vi "Initialize FPGA.vi"() -> (3 "IO Cluster Out":T1={"Error"={"status"=FALSE, "code"=0, "source"=""}, "Encoder Calibration Values"=[22, 216], "Update Calibration"=FALSE, "JPEG Resolutions"=3, "Raw Resolutions"=1, "Image Mode"=enum."RAW Gray Scale", "FPGA Ref"=refnum} {"JPEG Resolutions" items=["160x128"=3, "320x240"=5, "640x480"=7]; "Raw Resolutions" items=["80x60"=1, "160x120"=3, "128x128"=9, "128x96"=11]})   [LabVIEW 2019]
uses:
  QNET MS IO Cluster.ctl
  <vilib>/FPGAPlugInAG/myRIO-1900/niLvFpga_Open_myRIO-1900.vi
  <vilib>/rvi/interface/common/dynamic/niFpgaDynamicAddResources.vi
  <vilib>/rvi/interface/common/niFpgaWaitOnOcc.vi
  <vilib>/Utility/error.llb/Error Cluster From Error Code.vi
  <vilib>/rvi/errors/niLvFpgaAdjustHostInterfaceError.vi
  <vilib>/rvi/interface/nirviOpenFPGA/nirviOpenFPGA.xnode
  <vilib>/rvi/interface/nirviMethod/nirviMethod.xnode
  <vilib>/rvi/interface/nirviReadWriteControl/nirviReadWriteControl.xnode
  <vilib>/ErrorRing/Error Ring.xnode
  <vilib>/FPGAPlugInAG/Dynamic/niLvFpga_ConfigureFifo_Dynamic.vi
  <vilib>/rvi/errors/niLvFpgaMergeErrorWithErrorCode.vi
  <vilib>/FPGAPlugInAG/Dynamic/niLvFpga_StartFifo_Dynamic.vi
  NiFpgaLv.dll
  <vilib>/rvi/interface/Simulation/niFpgaSimulationCallBeginRW.vi
panel:
  out "Actual Depth":u32
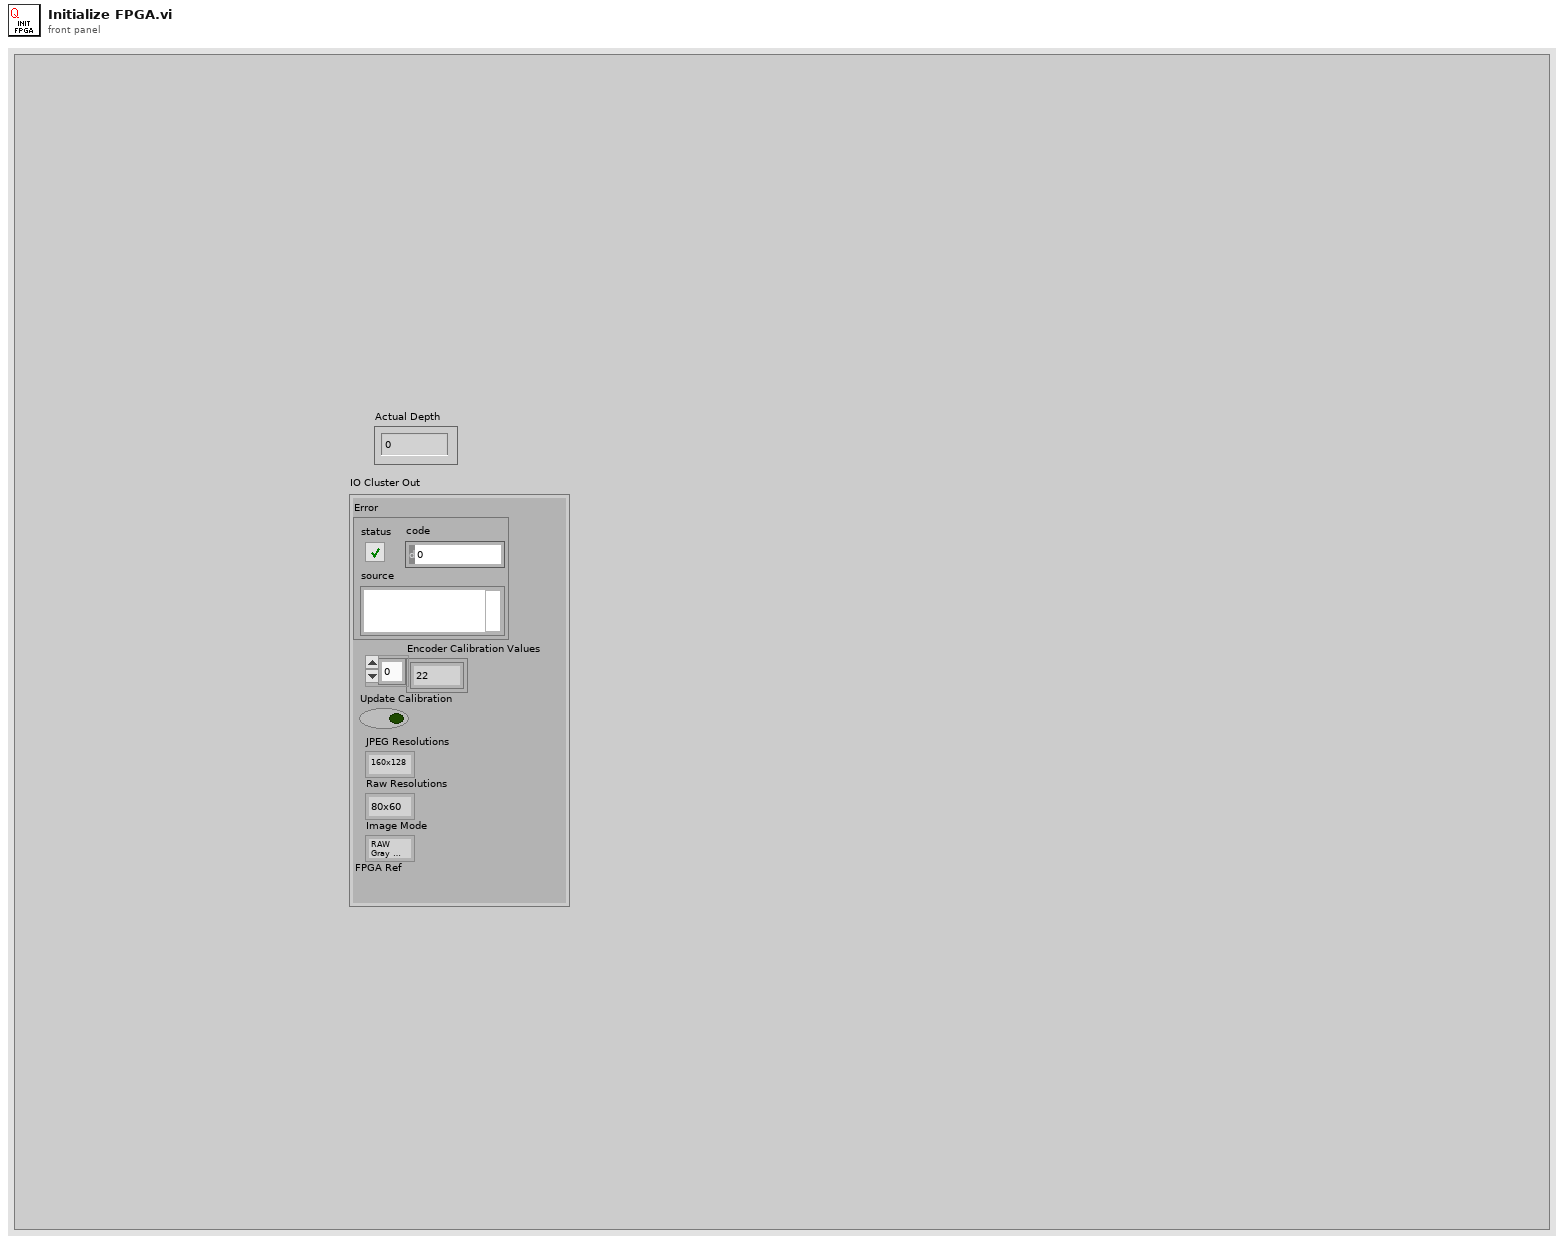
[diagram p1: front panel]
types:
  T1 = typedef "QNET MS IO Cluster.ctl" = cluster{"Error":errorcluster, "Encoder Calibration Values":i32[], "Update Calibration":bool, "JPEG Resolutions":u16, "Raw Resolutions":u16, "Image Mode":enum16{"RAW RGB", "RAW Gray Scale", "JPEG"}, "FPGA Ref":refnum<k20>}
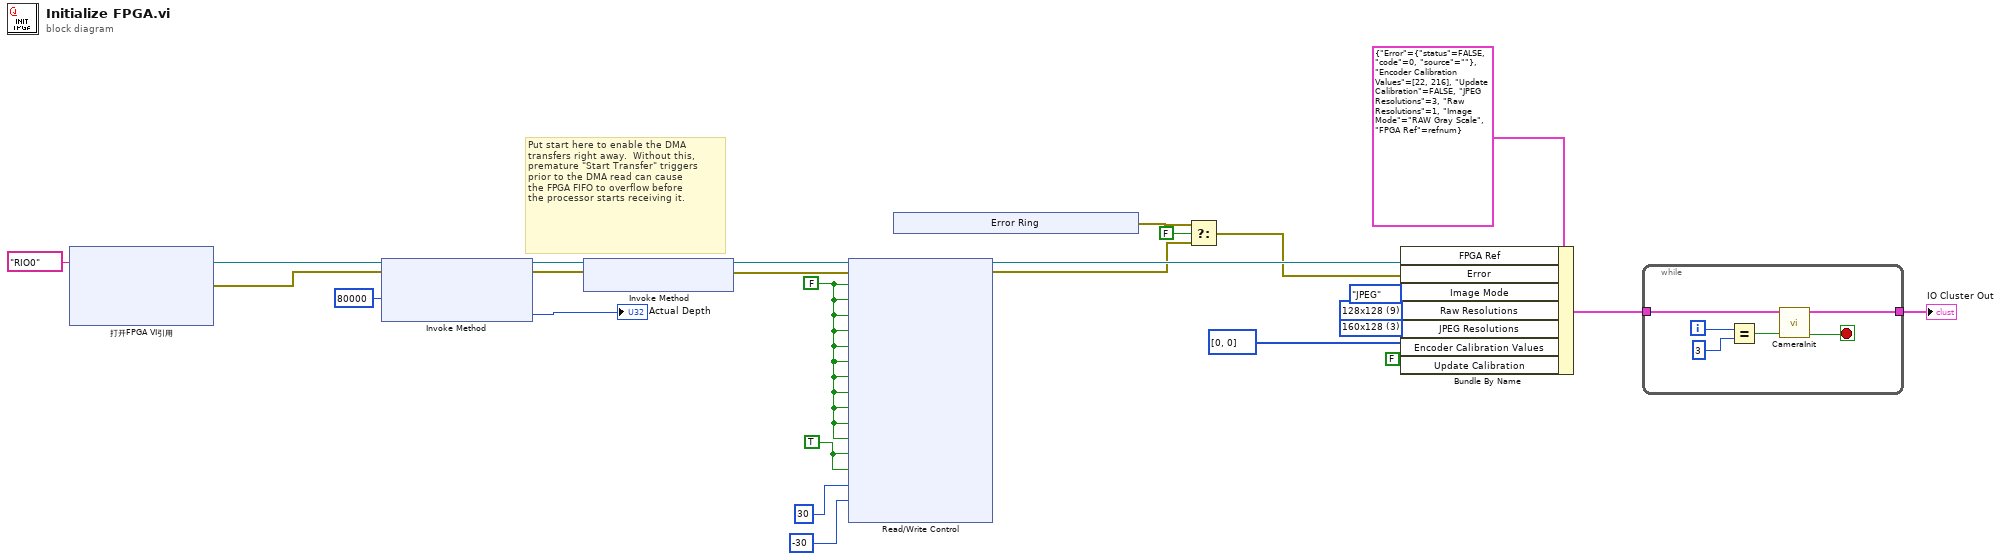
[diagram p0: block diagram]
diagram:
  w1 = TRUE ("PWM0 Enable")
  w4 = u16 3 items=["160x128"=3, "320x240"=5, "640x480"=7] ("JPEG Resolutions")
  w5 = u16 9 items=["80x60"=1, "160x120"=3, "128x128"=9, "128x96"=11] ("Raw Resolutions")
  w16 = FALSE ("PWM0 Enable")
  # "Put start here to enable the DMA\ntransfers right away.  Without this,\npremature \"Start Transfer\" triggers\nprior to the DMA read can cause\nthe FPGA FIFO to overflow before\nthe processor starts receiving it."
  n1 = xnode "打开FPGA VI引用"("资源名称"=tag "RIO0" ("resource name")) -> ("FPGA VI引用输出"=w20:refnum<k20>, "错误输出"=w26:errorcluster)  [unwired: 1 in]
  n2 = xnode "Invoke Method"("FPGA VI引用输入"=w20, "错误输入"=w26, "请求的深度"=u32 80000 ("Requested Depth")) -> ("FPGA VI引用输出"=w21:refnum<k20>, "错误输出"=w25:errorcluster, "实际深度"=→"Actual Depth":u32)
  n3 = xnode "Invoke Method"("FPGA VI引用输入"=w21, "错误输入"=w25) -> ("FPGA VI引用输出"=w19:refnum<k20>, "错误输出"=w18:errorcluster)
  n4 = xnode "Read/Write Control"("FPGA VI引用输入"=w19, "错误输入"=w18, "PWM0 Enable"=w16, "PWM1 Enable"=w16, "LED1 Red"=w16, "LED1 Yellow"=w16, "LED1 Green"=w16, "LED2 Red"=w16, "LED2 Yellow"=w16, "LED2 Green"=w16, "LED3 Red"=w16, "LED3 Yellow"=w16, "LED3 Green"=w16, "Encoder 0 Reset"=w1, "Encoder 1 Reset"=w1, "Encoder 0 Reset Value"=30, "Encoder 1 Reset Value"=-30) -> ("FPGA VI引用输出"=w17:refnum<k20>, "错误输出"=w12:errorcluster)  [unwired: 1 out]
  n5 = xnode "Error Ring"() -> ("错误输出"=w8:errorcluster)
  n6 = Select(t=w8, s=FALSE, f=w12) -> (s? t:f=w11:errorcluster)
  n7 = Bundle By Name(cluster=T1 {"Error"={"status"=FALSE, "code"=0, "source"=""}, "Encoder Calibration Values"=[22, 216], "Update Calibration"=FALSE, "JPEG Resolutions"=3, "Raw Resolutions"=1, "Image Mode"=enum."RAW Gray Scale", "FPGA Ref"=refnum} ("IO Cluster"), "FPGA Ref"=w17, "Error"=w11, "Image Mode"=enum16{"RAW RGB", "RAW Gray Scale", "JPEG"}."JPEG", "Raw Resolutions"=w5, "JPEG Resolutions"=w4, "Encoder Calibration Values"=i32[] [0, 0], "Update Calibration"=FALSE) -> (w13:T1)
  n8 = while {
    tunnel: w13 -> [w32]
    tunnel: [w27] -> w3
    i -> [w31]
    stop <- w29 stop-if-true
    n9 = Equal?(x=w31, y=3 ("x")) -> (x = y?=w28:bool)
    n10 = call "CameraInit.vi"("Last Attempt"=w28, "IO Cluster In"=w32) -> ("Exit"=w29:bool, "IO Cluster Out"=w27:T1)  [unwired: 6 in, 2 out]
  }
  "IO Cluster Out" <- w3
